vi "find best origin.vi"(11 "address":string) -> (3 "origin":string)   [LabVIEW 2016, in "websocket client.lvclass"]
uses:
  websocket client.lvclass
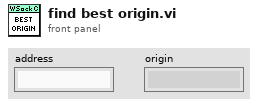
[diagram p1: front panel]
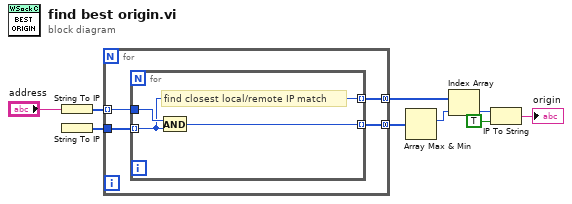
[diagram p0: block diagram]
diagram:
  n1 = String To IP(1:"address") -> (0:w4:u32[])
  n2 = String To IP() -> (0:w5:u32[])  [unwired: 1 in]
  n3 = for {
    tunnel: w4 -> [w12] mode=indexing
    tunnel: w5 -> [w13]
    tunnel: [w11] -> w6 mode=concatenating
    tunnel: [w10] -> w7 mode=concatenating
    n4 = for {
      tunnel: w13 -> [w14] mode=indexing
      tunnel: w12 -> [w16]
      tunnel: [w15] -> w11 mode=indexing
      tunnel: [w14] -> w10 mode=indexing
      # "find closest local/remote IP match"
      n5 = And(x=w16, y=w14) -> (x .and. y?=w15:u32)
    }
  }
  n6 = Array Max & Min(array=w6) -> (max index (indices)=w8:i32)  [unwired: 3 out]
  n7 = Index Array(array=w7, index=w8) -> (element=w9:u32)
  n8 = IP To String(1:TRUE ("dot notation? (F)"), 2:w9) -> (0:→"origin":string)
